vi "Find Setpoints in Dictionary.vi"(8 "error in (no error)":errorcluster, 9 "processing data dictionary":refnum<class "data dictionary.lvclass">, 10 "PID Loops in":refnum<class "PID Loop.lvclass">[](array[class]), 11 "Tagbus PID Module runtime":refnum<class "PID Module runtime.lvclass">) -> (0 "error out":errorcluster, 3 "Tagbus PID Module output":refnum<class "PID Module runtime.lvclass">)   [LabVIEW 2014, in "PID Module runtime.lvclass"]
uses:
  PID Module runtime.lvclass
  <vilib>/NI/Tag Bus/dictionary/data dictionary.lvclass
  configuration/PID Loop.lvclass
  <vilib>/NI/Tag Bus/tag/Data Type.ctl
  configuration/PID Loop/String Parameters.ctl
  PID Module runtime.lvclass/PID Module runtime.ctl
  <vilib>/NI/Tag Bus/tag/tag descriptor.lvclass
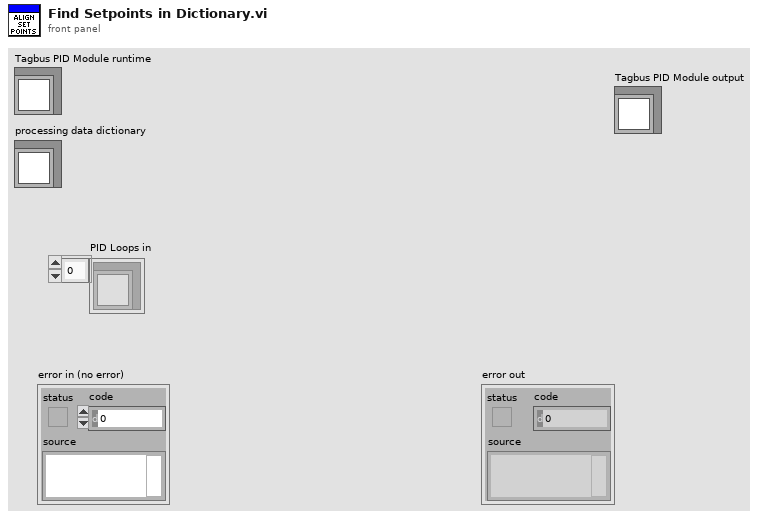
[diagram p1: front panel]
types:
  T1 = typedef "PID Loop.lvclass/String Parameters.ctl" = enum16{"Setpoint", "Process Variable", "Output", "Proportional Gain", "Integral Time", "Derivative Time", "Range High", "Range Low"}
  T2 = typedef "tag bus.lvlib/tag descriptor.lvclass/Data Type.ctl" = enum16{"Double", "Single", "I64", "I32", "I16", "I8", "U64", "U32", "U16", "U8", "Boolean", "String", "Array of Double", "Array of Single", "Array of I64", "Array of I32", "Array of I16", "Array of I8", "Array of U64", "Array of U32", "Array of U16", "Array of U8", "Array of Boolean", "Array of String"}
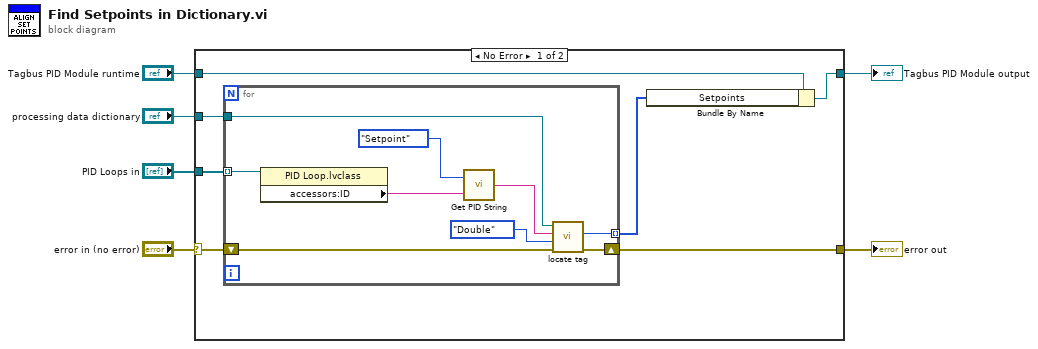
[diagram p0: block diagram]
diagram:
  n1 = case shown="No Error" "error in (no error)" {
    selector: "error in (no error)" -> [w11 w24]
    tunnel: [w10 w24] -> w5
    tunnel: "processing data dictionary" -> [w13 _]
    tunnel: "PID Loops in" -> [w12 _]
    tunnel: "Tagbus PID Module runtime" -> [w9 w23]
    tunnel: [w7 w23] -> w2
    frame No Error {
      n2 = for {
        tunnel: w13 -> [w22]
        tunnel: w12 -> [w17] mode=indexing
        shift-right: [w19] -> w10
        shift-left: w11 -> [w20]
        tunnel: [w18] -> w8 mode=indexing
        n3 = property class="PID Loop.lvclass"(reference=w17) -> ("accessors:ID"=w15:string)  [unwired: 1 in, 2 out]
        n4 = call "Get PID String.vi"("PID Loop ID"=w15, "PID Parameter"=String_Parameters."Setpoint") -> ("Parameter String"=w14:string)
        n5 = call <vilib>:"locate tag.vi"("error in"=w20, "data type"=Data_Type."Double", "name"=w14, "data dictionary in"=w22) -> ("error out"=w19:errorcluster, "index"=w18:i32)  [unwired: 5 in, 1 out]
      }
      n6 = Bundle By Name(cluster=w9, "Setpoints"=w8) -> (w7:refnum<class "PID Module runtime.lvclass">)
    }
    frame Error {
    }
  }
  "error out" <- w5
  "Tagbus PID Module output" <- w2
